vi "NMRvmeCard3Log.vi"() -> ()   [LabVIEW 2013]
uses:
  <vilib>/Utility/file.llb/Read From Spreadsheet File (DBL).vi
  <vilib>/Analysis/NI_AALBase.lvlib
panel:
  in  "Max":bool=TRUE
  in  "Logoffset (V)":dbl=-5.967500000000002 min=-9.0 max=9.0 step=0.0005 format="%_5g"
  in  "Phase (V)":dbl=6.5 min=0.0 max=9.0 step=0.0005 format="%_5g"
  out "Telnet error out":errorcluster
  in  "Real/Quad Q curve":bool=TRUE
  out "Temperature (C)":dbl(graph)=26.38
  out "+3V supply":dbl=3.245 format="%_4g"
  out "Temp (C)":dbl=26.38 format="%_4g"
  in  "RemovePed":bool=TRUE
  in  "IF / LOG Det":bool=TRUE
  in  "Q curve file":string="realback213.txt"
  out "File name 2":string="C:\\users\\plm\\Desktop\\rssmt\\realback213.txt"
  in  "AutoBaseline":bool
  out "RF OK":bool=TRUE
  out "Peak area (V-MHz)":sgl=0.0063264 format="%.5f"
  in  "Gauss Fit":bool
  out "NMR Graph + Fit":cluster{cluster{dbl, "Numeric":dbl}[]}[](graph)=[{[{212.6, "Numeric"=-0.0589791666666753}, {212.60999999999999, "Numeric"=-0.004679166666739676}, {212.62, "Numeric"=0.022620833333395873}, {212.63, "Numeric"=0.024720833333333025}, {212.64, "Numeric"=0.03202083333327316}, {212.65, "Numeric"=0.04862083333339834}, {212.66, "Numeric"=0.029720833333340024}, {212.67, "Numeric"=0.011720833333285163}, {212.68, "Numeric"=0.006820833333399612}, {212.69, "Numeric"=-0.004579166666654089}, {212.7, "Numeric"=0.07552083333329557}, {212.71, "Numeric"=0.03572083333339954}, {212.72, "Numeric"=0.04322083333335064}, {212.73, "Numeric"=0.02442083333330508}, {212.74, "Numeric"=-0.005379166666737378}, {212.75, "Numeric"=0.04212083333335409}, {212.76, "Numeric"=0.03572083333331316}, {212.77, "Numeric"=0.011720833333275449}, {212.78, "Numeric"=0.09272083333335629}, {212.79, "Numeric"=0.015620833333320094}, {212.8, "Numeric"=-0.01927916666671281}, {212.81, "Numeric"=0.011320833333357205}, {212.82, "Numeric"=0.0721208333333258}, {212.82999999999998, "Numeric"=0.0054208333332975145}, {212.84, "Numeric"=0.05942083333335696}, {212.85, "Numeric"=0.05652083333333016}, {212.85999999999999, "Numeric"=0.08162083333330661}, {212.87, "Numeric"=0.06572083333335546}, {212.88, "Numeric"=0.0642208333333334}, {212.89, "Numeric"=0.09962083333331456}, {212.9, "Numeric"=0.011420833333352753}, {212.91, "Numeric"=0.040520833333335365}, {212.92, "Numeric"=0.010220833333321244}, {212.93, "Numeric"=0.020920833333348765}, {212.94, "Numeric"=0.055520833333336045}, {212.95, "Numeric"=0.017320833333326652}, {212.96, "Numeric"=0.039420833333343536}, {212.97, "Numeric"=0.12312083333333557}, {212.98, "Numeric"=0.17172083333333088}, {212.99, "Numeric"=0.14202083333332943}, {213.0, "Numeric"=0.08832083333333385}, {213.01, "Numeric"=0.02572083333333383}, {213.02, "Numeric"=0.005220833333337116}, {213.03, "Numeric"=0.03162083333333085}, {213.04, "Numeric"=-0.029979166666664434}, {213.05, "Numeric"=-0.01657916666665646}, {213.06, "Numeric"=0.06442083333332665}, {213.07, "Numeric"=0.009120833333336048}, {213.08, "Numeric"=-0.04317916666665124}, {213.09, "Numeric"=-0.012379166666678765}, {213.1, "Numeric"=-0.12677916666666467}, {213.11, "Numeric"=-0.13277916666664727}, {213.12, "Numeric"=-0.15497916666668543}, {213.13, "Numeric"=-0.18697916666666664}, {213.14000000000001, "Numeric"=-0.030079166666644536}, {213.15, "Numeric"=-0.03087916666669338}, {213.16, "Numeric"=-0.029879166666669815}, {213.17000000000002, "Numeric"=-0.03347916666664302}, {213.18, "Numeric"=-0.006079166666702496}, {213.19, "Numeric"=0.0014208333333257661}, {213.2, "Numeric"=-0.015679166666642763}, {213.21, "Numeric"=-0.026579166666712895}, {213.22, "Numeric"=-0.04657916666667994}, {213.23, "Numeric"=-0.023279166666643814}, {213.24, "Numeric"=-0.04307916666660422}, {213.25, "Numeric"=-0.04667916666668687}, {213.26, "Numeric"=-0.020979166666645954}, {213.27, "Numeric"=-0.015279166666601729}, {213.28, "Numeric"=-0.03447916666669487}, {213.29, "Numeric"=-0.022179166666649375}, {213.3, "Numeric"=-0.03607916666660044}, {213.31, "Numeric"=-0.025179166666704333}, {213.32, "Numeric"=-0.024979166666654062}, {213.33, "Numeric"=-0.052779166666600486}, {213.34, "Numeric"=-0.05967916666671497}, {213.35, "Numeric"=-0.024279166666660024}, {213.36, "Numeric"=0.009920833333398382}, {213.37, "Numeric"=-0.015479166666726718}, {213.38, "Numeric"=-0.004279166666667111}, {213.39000000000001, "Numeric"=-0.02427916666660429}, {213.4, "Numeric"=0.0410208333332604}]}]
  in  "Amp of Q curve":dbl=9.000000000000004 min=0.0 max=10.0 step=0.01 format="%_3f"
  in  "Subtract Q curve":bool=TRUE
  in  "Adjust Tune":bool
  out "Pedestal Offset":dbl(graph)=0.15075416666666658
  out "Pedestal Difference":dbl(graph)=-0.04574999999998802
  out "# Good Spectra":i32=94
  in  "Quality cuts":bool=TRUE
  out "Pedestal OK":bool=TRUE
  out "Sweep #":i32=4061
  out "1st Sweep":bool
  out "ADC volts OK":bool=TRUE
  out "Peak Height Distribution":cluster{"Y":dbl[], "Y":dbl[]}[](graph)=[{"Y"=[0.2602259791666628, 0.2626737708333295, 0.26512156249999613, 0.2675693541666628, 0.2700171458333295, 0.2724649374999961, 0.2749127291666628, 0.27736052083332946, 0.2798083124999961, 0.2822561041666628, 0.28470389583332945, 0.28715168749999614, 0.2895994791666628, 0.2920472708333295, 0.29449506249999613, 0.2969428541666628, 0.29939064583332947, 0.3018384374999961, 0.3042862291666628, 0.30673402083332946, 0.3091818124999961, 0.3116296041666628, 0.31407739583332944, 0.31652518749999614, 0.3189729791666628, 0.32142077083332943, 0.3238685624999961, 0.32631635416666277, 0.32876414583332947, 0.3312119374999961, 0.3336597291666628, 0.33610752083332945, 0.3385553124999961, 0.3410031041666628, 0.34345089583332944, 0.34589868749999614, 0.3483464791666628, 0.3507942708333294, 0.3532420624999961, 0.35568985416666277, 0.35813764583332947, 0.3605854374999961, 0.36303322916666275, 0.36548102083332945, 0.3679288124999961, 0.3703766041666628, 0.37282439583332944, 0.3752721874999961, 0.3777199791666628, 0.3801677708333294, 0.3826155624999961, 0.38506335416666276, 0.38751114583332946, 0.3899589374999961, 0.39240672916666275, 0.39485452083332945, 0.3973023124999961, 0.3997501041666628, 0.40219789583332943, 0.4046456874999961, 0.4070934791666628, 0.4095412708333294, 0.4119890624999961, 0.41443685416666276, 0.4168846458333294, 0.4193324374999961, 0.42178022916666275, 0.42422802083332944, 0.4266758124999961, 0.4291236041666628, 0.43157139583332943, 0.4340191874999961, 0.43646697916666277, 0.4389147708333294, 0.4413625624999961, 0.44381035416666276, 0.4462581458333294, 0.4487059374999961, 0.45115372916666274, 0.45360152083332944, 0.4560493124999961, 0.45849710416666273, 0.4609448958333294, 0.46339268749999607, 0.46584047916666277, 0.4682882708333294, 0.47073606249999606, 0.47318385416666275, 0.4756316458333294, 0.4780794374999961, 0.48052722916666274, 0.48297502083332944, 0.4854228124999961, 0.4878706041666627, 0.4903183958333294, 0.49276618749999607, 0.49521397916666277, 0.4976617708333294, 0.500109562499996, 0.5025573541666627], "Y"=[2.0, 0.0, 0.0, 0.0, 1.0, 1.0, 0.0, 0.0, 0.0, 1.0, 0.0, 0.0, 0.0, 1.0, 3.0, 0.0, 0.0, 3.0, 2.0, 1.0, 0.0, 0.0, 2.0, 1.0, 1.0, 0.0, 1.0, 1.0, 2.0, 0.0, 2.0, 2.0, 3.0, 2.0, 3.0, 0.0, 3.0, 0.0, 2.0, 0.0, 2.0, 2.0, 1.0, 1.0, 2.0, 2.0, 1.0, 3.0, 2.0, 2.0, 2.0, 3.0, 1.0, 0.0, 0.0, 2.0, 1.0, 2.0, 0.0, 5.0, 0.0, 2.0, 3.0, 0.0, 2.0, 2.0, 1.0, 0.0, 0.0, 1.0, 1.0, 0.0, 1.0, 0.0, 0.0, 0.0, 0.0, 1.0, 1.0, 0.0, 0.0, 0.0, 0.0, 0.0, 0.0, 1.0, 0.0, 0.0, 0.0, 0.0, 1.0, 1.0, 1.0, 0.0, 0.0, 0.0, 0.0, 0.0, 0.0, 1.0]}]
  in  "# of Sweeps":i32=10000
  out "S/N":dbl=7.010209139899895 format="%_3g"
  out "Peak mean (V)":dbl=0.3667999335106349 format="%_4g"
  out "Peak Height":dbl(graph)=0.17172083333333088
  in  "Raw Data":bool=TRUE
  in  "Tank RF":bool=TRUE
  in  "IF Atten (dB)":i8=4 min=0 max=31 step=1
  in  "IFoffset (V)":dbl=6.090664000000002 min=-0.0 max=9.0 step=0.001 format="%.4f"
  in  "Tune  (V)":dbl=1.4152000000000005 min=-0.5 max=5.0 step=0.001 format="%.4f"
  in  "Hi / Lo Gain":bool
  out "Voltage Array":sgl[](array[numeric])=[1.568, 1.5503, 1.5074, 1.4411, 1.3818, 1.3336, 1.2517, 1.1725, 1.1082, 1.0392, 1.0635, 0.9697, 0.925, 0.8558, 0.7774, 0.7781, 0.7267, 0.6595, 0.6991, 0.5824, 0.5097, 0.5043, 0.5309, 0.4318, 0.4552, 0.4235, 0.4216, 0.3805, 0.3556, 0.3694, 0.2614, 0.2725, 0.226, 0.2223, 0.2443, 0.1953, 0.2084, 0.2849, 0.3281, 0.2948, 0.2393, 0.1767, 0.158, 0.188, 0.1318, 0.1524, 0.2424, 0.1979, 0.1582, 0.2034, 0.1052, 0.1172, 0.1148, 0.1044, 0.2847, 0.3091, 0.3371, 0.3623, 0.4203, 0.4602, 0.4773, 0.5024, 0.5202, 0.5831, 0.6047, 0.6443, 0.715, 0.7675, 0.7969, 0.8596, 0.8979, 0.9628, 1.0188, 1.0486, 1.1011, 1.1977, 1.2949, 1.3343, 1.4121, 1.4605, 1.596] format="%.4f"
  in  "Invert Polarity":bool
  out "Pedestal Diff (V)":sgl=-0.04575 format="%.3f"
  out "Peak amp (V)":sgl=0.17172083 format="%.3f"
  in  "Save Data to File":bool
  in  "RF Level (dBm)":dbl min=-10.0 max=10.0 step=0.1 format="%.2f"
  out "SMT error out":errorcluster
  out "Sample RMS (V)":dbl=0.013479012345679013 format="%.4f"
  in  "# Sample/step":i32=80 min=1 max=1000 step=100
  in  "Step Width (MHz)":dbl=0.01 min=0.0 max=1000.0 step=0.0005 format="%.4f"
  in  "Freq Span (MHz)":dbl=0.8 min=0.0 max=3000.0 step=0.1 format="%.3f"
  in  "Center Freq (MHz)":dbl=213.0 min=0.005 max=6000.0 step=0.1 format="%.3f"
  in  "Sweep Mode":u16(ring)=3 items=["Off", "Single", "Auto", "Step"]
  in  "GPIB Addr (28)":refnum<visa-resource-name>="GPIB0::28::INSTR"
  # "E1039 Prototype NMR Control Panel"
  # "Settings"
  # "D\nA\nC"
  # "R\nF\n\nG\nE\nN \n\n+\n\nI\nF"
  # "A\nD\nC"
  # "I\n/\nO"
  # "D\nA\nT\nA\n\nA \nN\nA\nL\nY\nS\nI\nS"
  # "Results"
  # "A\nv\ne\nr\na\ng\ne"
  # "S\nw\ne\ne\np"
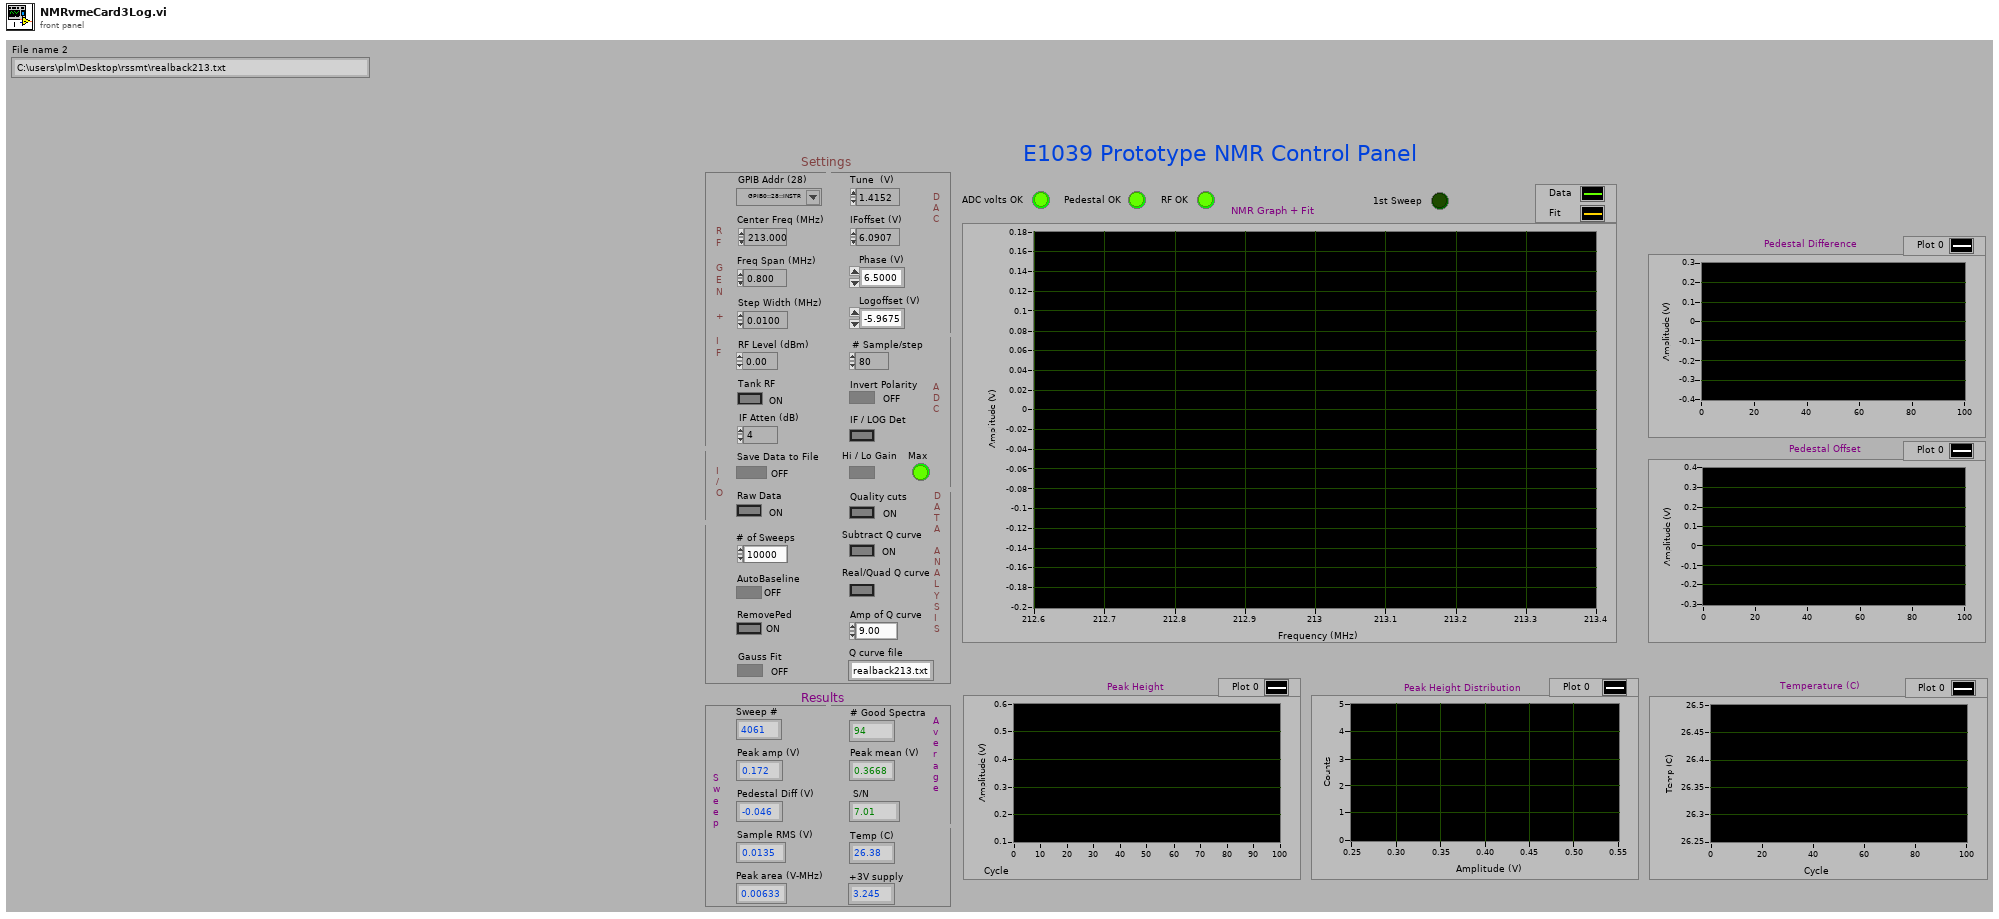
[diagram p1: front panel]
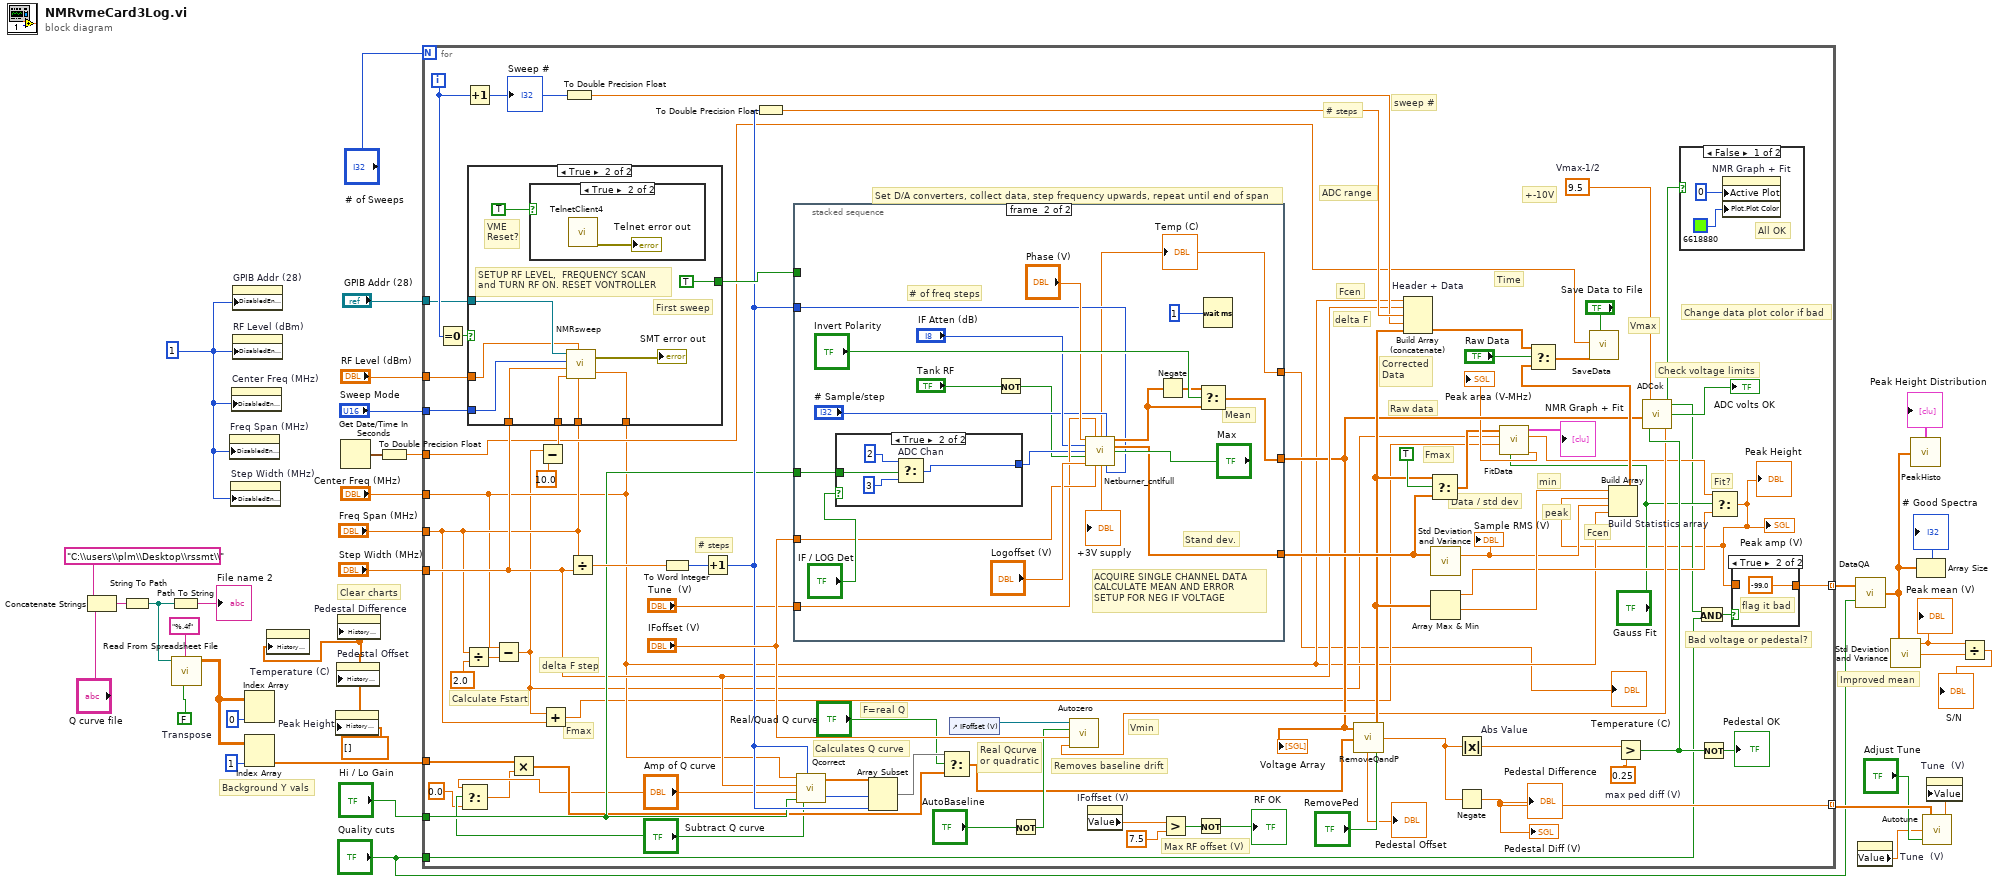
[diagram p0: block diagram]
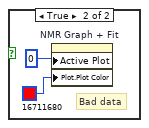
[diagram p2: hidden frame]
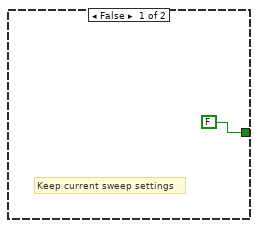
[diagram p4: hidden frame]
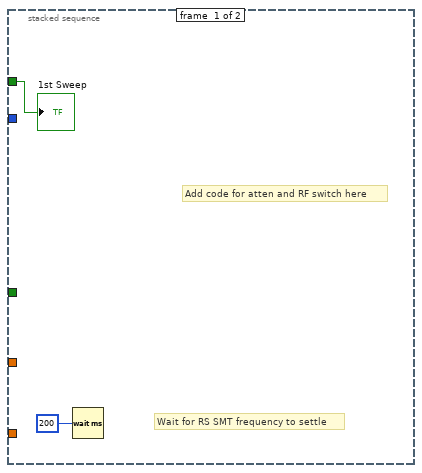
[diagram p6: hidden frame]
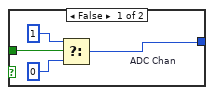
[diagram p7: hidden frame]
diagram:
  w1 = 1
  w13 = FALSE  # Transpose
  w5 = dbl[] []
  # "Background Y vals"
  # "Clear charts"
  # "Improved mean"
  n1 = Concatenate Strings "Concatenate Strings"("C:\\users\\plm\\Desktop\\rssmt\\", "Q curve file") -> (w16:string)
  n2 = String To Path(string=w16) -> (path=w12:path)
  n3 = Path To String(path=w12) -> (string=→"File name 2":string)
  n4 = call-poly <vilib>:"Read From Spreadsheet File.vi"("transpose (no:F)"=w13, "format (%.3f)"="%.4f", "file path (dialog if empty)"=w12) -> ("all rows"=w11:dbl[][])  [unwired: 4 in, 4 out]
  n5 = property on="Freq Span (MHz)" class="DigNum (strict)"("DisabledEnum"=w1) -> ()  [unwired: 2 in, 2 out]
  n6 = property on="Step Width (MHz)" class="DigNum (strict)"("DisabledEnum"=w1) -> ()  [unwired: 2 in, 2 out]
  n7 = property on="Center Freq (MHz)" class="DigNum (strict)"("DisabledEnum"=w1) -> ()  [unwired: 2 in, 2 out]
  n8 = property on="GPIB Addr (28)" class="VISAName"("DisabledEnum"=w1) -> ()  [unwired: 2 in, 2 out]
  n9 = property on="RF Level (dBm)" class="DigNum (strict)"("DisabledEnum"=w1) -> ()  [unwired: 2 in, 2 out]
  n10 = Index Array "Index Array"(array=w11, index (col)=0) -> ()  [unwired: 1 in, 1 out]
  n11 = Index Array(array=w11, index (col)=1) -> (element=w6:dbl[])  [unwired: 1 in]
  n12 = property on="Temperature (C)" class="WFChart (strict)"("History Data"=w5) -> ()  [unwired: 2 in, 2 out]
  n13 = property on="Peak Height" class="WFChart (strict)"("History Data"=w5) -> ()  [unwired: 2 in, 2 out]
  n14 = property on="Pedestal Offset" class="WFChart (strict)"("History Data"=w5) -> ()  [unwired: 2 in, 2 out]
  n15 = property on="Pedestal Difference" class="WFChart (strict)"("History Data"=w5) -> ()  [unwired: 2 in, 2 out]
  n16 = Get Date/Time In Seconds() -> (seconds since 1Jan1904=w18:timestamp)
  n17 = To Double Precision Float(number=w18) -> (double precision float=w17:dbl)
  n18 = for {
    N: "# of Sweeps" -> [_]
    tunnel: [w96] -> w33 mode=indexing
    tunnel: "Quality cuts" -> [w73]
    tunnel: [w79] -> w30 mode=indexing
    tunnel: "Center Freq (MHz)" -> [w60]
    tunnel: "Freq Span (MHz)" -> [w66]
    tunnel: "Step Width (MHz)" -> [w72]
    tunnel: "Sweep Mode" -> [w83]
    tunnel: "Hi / Lo Gain" -> [w82]
    tunnel: "GPIB Addr (28)" -> [w81]
    tunnel: "RF Level (dBm)" -> [w80]
    tunnel: w17 -> [w67]
    tunnel: w6 -> [w45]
    i -> [w94]
    w77 = 9.5  # Vmax-1/2
    w97 = 0.25  # max ped diff (V)
    # "F=real Q"
    # "Real Qcurve\nor quadratic"
    # "+-10V"
    # "Vmax"
    # "Change data plot color if bad"
    # "Max RF offset (V)"
    # "Fmax"
    # "Fit?"
    # "Fmax"
    # "Time"
    # "Vmin"
    # "min"
    # "peak"
    # "Raw data"
    # "Corrected\nData"
    # "Fcen"
    # "delta F"
    # "# steps"
    # "ADC range"
    # "sweep #"
    # "Fcen"
    # "Set D/A converters, collect data, step frequency upwards, repeat until end of span"
    # "Calculates Q curve"
    # "Removes baseline drift"
    # "Bad voltage or pedestal?"
    # "Check voltage limits"
    # "Data / std dev"
    # "# steps"
    # "Calculate Fstart"
    # "delta F step"
    n19 = Equal To 0?(x=w94) -> (x = 0?=w99:bool)
    n20 = Select(t="Amp of Q curve", s="Subtract Q curve", f=0.0) -> (s? t:f=w40:dbl)
    n21 = Divide(x=w66, y=sgl 2.0) -> (x/y=w110:dbl)
    n22 = Increment(x=w94) -> (x+1=w84:i32)
    "Sweep #" <- w84
    n23 = Subtract(x=w60, y=w110) -> (x-y=w55:dbl)
    n24 = Multiply(x=w45, y=w40) -> (x*y=w44:dbl[])
    n25 = Subtract(x=w55, y=10.0) -> (x-y=w108:dbl)
    n26 = case shown="True" w99 {
      tunnel: w108 -> [_ w129]
      tunnel: w72 -> [_ w127]
      tunnel: w60 -> [_ w126]
      tunnel: w66 -> [_ w128]
      tunnel: [FALSE TRUE] -> w98
      tunnel: w83 -> [_ w123]
      tunnel: w81 -> [_ w122]
      tunnel: w80 -> [_ w121]
      frame False {
        # "Keep current sweep settings"
      }
      frame True {
        # "VME\nReset?"
        # "First sweep"
        # "SETUP RF LEVEL,  FREQUENCY SCAN\nand TURN RF ON. RESET VONTROLLER"
        n27 = case shown="True" TRUE {
          frame False {
          }
          frame True {
            n28 = call "TelnetClient4.vi"() -> ("Telnet error"=→"Telnet error out":errorcluster)  [unwired: 4 in, 3 out]
          }
        }
        n29 = call "NMRsweep.vi"("Center Freq (MHz)"=w126, "Freq Span (MHz)"=w128, "RF Level (dBm)"=w121, "Foffset (MHz)"=w129, "Step Width (MHz)"=w127, "Sweep Mode"=w123, "GPIB Addr (28)"=w122) -> ("error out"=→"SMT error out":errorcluster)
      }
    }
    n30 = Add(x=w55, y=w66) -> (x+y=w54:dbl)
    n31 = To Double Precision Float(number=w84) -> (double precision float=w85:dbl)
    n32 = Divide(x=w66, y=w72) -> (x/y=w112:dbl)
    n33 = To Word Integer(number=w112) -> (16bit integer=w109:i16)
    n34 = Increment(x=w109) -> (x+1=w88:i16)
    n35 = To Double Precision Float(number=w88) -> (double precision float=w87:dbl)
    n36 = stacked-sequence {
      tunnel: [_ w140] -> w102
      tunnel: [_ w151] -> w70
      tunnel: w88 -> [_ w137]
      tunnel: "IFoffset (V)" -> [_ w146]
      tunnel: w82 -> [_ w149]
      tunnel: w98 -> [w131 _]
      tunnel: "Tune  (V)" -> [_ w144]
      tunnel: [_ w135] -> w36
      frame #0 {
        # "Add code for atten and RF switch here"
        # "Wait for RS SMT frequency to settle"
        n37 = Wait (ms)(milliseconds to wait=200) -> ()  [unwired: 1 out]
        "1st Sweep" <- w131
      }
      frame #1 {
        # "Stand dev."
        # "Mean"
        # "ACQUIRE SINGLE CHANNEL DATA\nCALCULATE MEAN AND ERROR\nSETUP FOR NEG IF VOLTAGE"
        # "# of freq steps"
        n38 = case shown="True" "IF / LOG Det" {
          tunnel: w149 -> [w157 w158]
          tunnel: [w154 w159] -> w139
          frame False {
            n39 = Select "ADC Chan"(t=1, s=w157, f=0) -> (s? t:f=w154:i32)
          }
          frame True {
            n40 = Select "ADC Chan"(t=2, s=w158, f=3) -> (s? t:f=w159:i32)
          }
        }
        n41 = Not(x="Tank RF") -> (.not. x?=w134:bool)
        n42 = call "Netburner_cntlfull.vi"("Phase Volt"="Phase (V)", "Tune Volt"=w144, "# Data"="# Sample/step", "IF Atten (dB)"="IF Atten (dB)", "NMR ADC"=w139, "Hi Gain"="Max", "Tank RF"=w134, "LogOff Volt"="Logoffset (V)", "IFOff Volt"=w146, "# f steps"=w137) -> ("Temp (C)"=w135:dbl, "ADC value"=w141:dbl[], "ADC error"=w140:dbl[], "Volts"=→"+3V supply":dbl)  [unwired: 2 out]
        "Temp (C)" <- w135
        n43 = Negate(x=w141) -> (-x=w150:dbl[])
        n44 = Select(t=w150, s="Invert Polarity", f=w141) -> (s? t:f=w151:dbl[])
        n45 = Wait (ms)(milliseconds to wait=1) -> ()  [unwired: 1 out]
      }
    }
    "Voltage Array" <- w70
    "Temperature (C)" <- w36
    n46 = call "Qcorrect.vi"("Subtract Q curve"="Subtract Q curve", "Nstep"=w88, "IF or Log"=w82, "Amp of Q curve"="Amp of Q curve", "Step Width (MHz)"=w72, "Center Freq (MHz)"=w60) -> ("Start"=w103:i32, "Array"=w104:dbl[])
    n47 = Array Subset "Array Subset"(array=w104, index=w103, length=w88) -> (w48:dbl[])
    n48 = Select(t=w48, s="Real/Quad Q curve", f=w44) -> (s? t:f=w47:dbl[])
    n49 = control-ref of="IFoffset (V)"() -> (w76:refnum<vi>)
    n50 = Not(x="AutoBaseline") -> (.not. x?=w49:bool)
    n51 = property on="IFoffset (V)" class="DigNum (strict)"() -> ("Value"=w64:dbl)  [unwired: 2 in, 2 out]
    n52 = Greater?(x=w64, y=7.5) -> (0:w62:bool)
    n53 = Not(x=w62) -> (.not. x?=→"RF OK":bool)
    n54 = call "RemoveQandP.vi"("Subtract Ped?"="RemovePed", "Qcurve"=w47, "Raw data"=w70) -> ("Ped L-R"=w90:dbl, "Corrected data"=w86:dbl[], "Ped Offfset"=→"Pedestal Offset":dbl)
    n55 = Build Array (concatenate) "Header + Data"(w60, w72, w87, w85, w86) -> (w89:dbl[])
    n56 = Select(t=w86, s=TRUE, f=w102) -> (s? t:f=w56:dbl[])
    n57 = call <vilib>:"Std Deviation and Variance.vi"("X"=w102) -> ("mean"=w71:dbl)  [unwired: 1 in, 2 out]
    "Sample RMS (V)" <- w71
    n58 = Array Max & Min(array=w86) -> (max value=w65:dbl, min value=w101:dbl)  [unwired: 2 out]
    n59 = Absolute Value "Abs Value"(x=w90) -> (abs(x)=w92:dbl)
    n60 = Negate(x=w90) -> (-x=w79:dbl)
    "Pedestal Diff (V)" <- w79
    "Pedestal Difference" <- w79
    n61 = call "FitData.vi"("Fit?"="Gauss Fit", "Fmax"=w54, "Fmin"=w55, "Yarray"=w56) -> ("Peak Area (V-MHz)"=→"Peak area (V-MHz)":dbl, "Amplitude (V)"=w58:dbl, "NMR Graph + Fit"=→"NMR Graph + Fit":cluster{cluster{dbl, "Numeric":dbl}[]}[])  [unwired: 2 out]
    n62 = Greater?(x=w92, y=w97) -> (0:w78:bool)
    n63 = call "ADCok.vi"("PedOK"=w78, "Array"=w70, "Vmax-1/2"=w77) -> ("Vmin"=w75:dbl, "ADC voltages OK"=→"ADC volts OK":bool, "Allok"=w52:bool)
    n64 = call "Autozero.vi"("Vmin (V)"=w75, "IFoffset (V)"="IFoffset (V)", "IF or Log"=w49, "reference"=w76) -> ()
    n65 = case shown="False" w52 {
      frame False {
        # "All OK"
        n66 = property on="NMR Graph + Fit" class="XYGraph (strict)"("Active Plot"=0, "Plot.Plot Color"=u32 6618880) -> ()  [unwired: 2 in, 2 out]
      }
      frame True {
        # "Bad data"
        n67 = property on="NMR Graph + Fit" class="XYGraph (strict)"("Active Plot"=0, "Plot.Plot Color"=u32 16711680) -> ()  [unwired: 2 in, 2 out]
      }
    }
    n68 = And(x=w52, y=w73) -> (x .and. y?=w93:bool)
    n69 = Not(x=w78) -> (.not. x?=→"Pedestal OK":bool)
    n70 = Select(t=w58, s="Gauss Fit", f=w65) -> (s? t:f=w51:dbl)
    "Peak amp (V)" <- w51
    "Peak Height" <- w51
    n71 = Build Array "Build Statistics array"(w101, w51, w71, w60) -> (w107:dbl[])
    n72 = Select(t=w89, s="Raw Data", f=w107) -> (s? t:f=w68:dbl[])
    n73 = call "SaveData.vi"("Array"=w68, "Save Data to File"="Save Data to File", "Ext time (sec)"=w67) -> ()  [unwired: 1 out]
    n74 = case shown="True" w93 {
      tunnel: [w117 -99.0] -> w96
      tunnel: w51 -> [w117 _]
      frame False {
        # "Data OK"
      }
      frame True {
        # "flag it bad"
      }
    }
  }
  n75 = call "DataQA.vi"("Quality cuts"="Quality cuts", "Data In"=w33) -> ("Data Out"=w32:dbl[])
  n76 = property on="Tune  (V)" class="DigNum (strict)"() -> ("Value"=w21:dbl)  [unwired: 2 in, 2 out]
  n77 = call <vilib>:"Std Deviation and Variance.vi"("X"=w32) -> ("mean"=w4:dbl, "standard deviation"=w3:dbl)  [unwired: 1 in, 1 out]
  "Peak mean (V)" <- w4
  n78 = call "PeakHisto.vi"("Data Out"=w32) -> ("XY Graph"=→"Peak Height Distribution":cluster{"Y":dbl[], "Y":dbl[]}[])
  n79 = Array Size(array=w32) -> (size(s)=→"# Good Spectra":i32)
  n80 = call "Autotune.vi"("Adjust Tune"="Adjust Tune", "Tune Vin"=w21, "Pedestal Diff"=w30) -> ("Tune Vout"=w20:dbl)
  n81 = property on="Tune  (V)" class="DigNum (strict)"("Value"=w20) -> ()  [unwired: 2 in, 2 out]
  n82 = Divide(x=w4, y=w3) -> (x/y=→"S/N":dbl)
